vi "Start New File.vi"(8 "error in":errorcluster, 11 "GUI Facade in":refnum<class "GUI Facade.lvclass">) -> (0 "error out":errorcluster, 3 "GUI Facade out":refnum<class "GUI Facade.lvclass">)   [LabVIEW 2018, in "GUI Facade.lvclass"]
uses:
  GUI Facade.lvclass
  File IO/Class/File Observer.lvclass
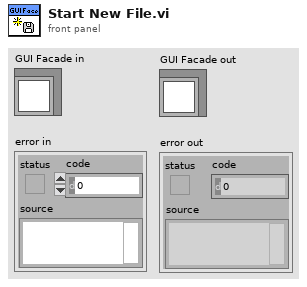
[diagram p1: front panel]
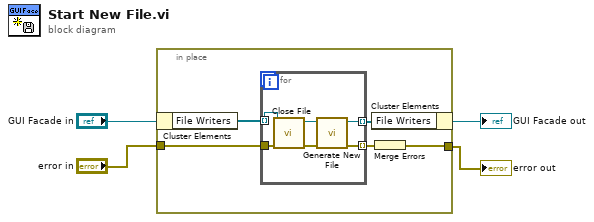
[diagram p0: block diagram]
diagram:
  n1 = in-place {
    in-place-border: "error in" -> [w7]
    in-place-border: [w5] -> w2
    n2 = in-place-cluster #1("GUI Facade in") -> ("File Writers"=w9:refnum<class "File Observer.lvclass">[])
    n3 = for {
      tunnel: w9 -> [w15] mode=indexing
      tunnel: [w13] -> w8 mode=indexing
      tunnel: w7 -> [w12]
      tunnel: [w11] -> w6 mode=indexing
      n4 = call-dynamic "Close File.vi"("error in"=w12, "File Obs in"=w15) -> ("error out"=w10:errorcluster, "File Obs out"=w14:refnum<class "File Observer.lvclass">)  [unwired: 8 in]
      n5 = call-dynamic "Generate New File.vi"("error in"=w10, "File Obs in"=w14) -> ("error out"=w11:errorcluster, "File Obs out"=w13:refnum<class "File Observer.lvclass">)  [unwired: 7 in, 1 out]
    }
    n6 = in-place-cluster #1("File Writers"=w8) -> (→"GUI Facade out":refnum<class "GUI Facade.lvclass">)
    n7 = Merge Errors(w6) -> (w5:errorcluster)
  }
  "error out" <- w2
